vi "Init.vi"(8 "error in (no error)":errorcluster, 9 "Config File Path":path=path "", 10 "Name":string, 11 "Base In":refnum<class "Base.lvclass">) -> (0 "error out":errorcluster, 3 "Base Out":refnum<class "Base.lvclass">)   [LabVIEW 2020, in "Base.lvclass"]
doc: "Initialize the class and creates necessary references. Anything initialized here is released in the Clear.vi method."
uses:
  Base.lvclass
  Base.lvclass/Base.ctl
  <vilib>/Utility/file.llb/Application Directory.vi
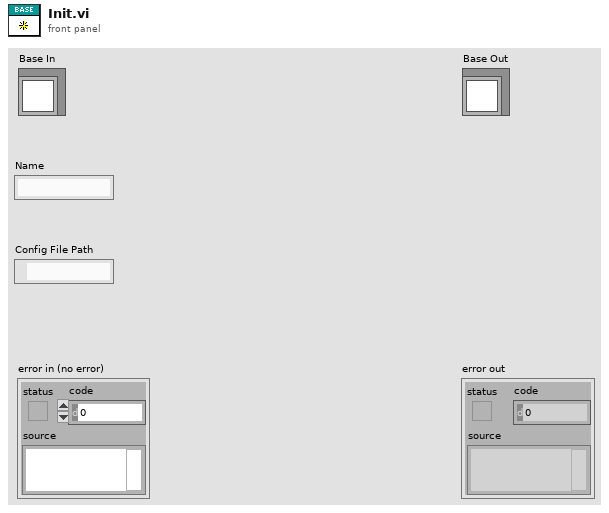
[diagram p1: front panel]
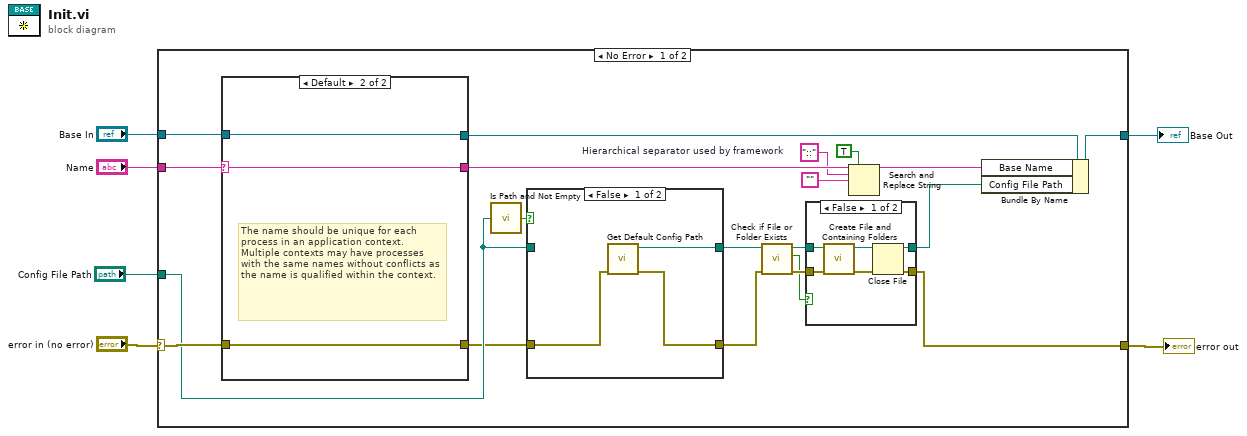
[diagram p0: block diagram]
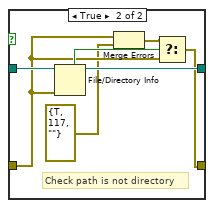
[diagram p3: hidden frame]
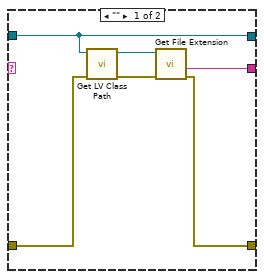
[diagram p4: hidden frame]
diagram:
  n1 = case shown="No Error" "error in (no error)" {
    selector: "error in (no error)" -> [w22 w54]
    tunnel: [w26 w55] -> w6
    tunnel: "Base In" -> [w25 w55]
    tunnel: "Name" -> [w23 _]
    tunnel: "Config File Path" -> [w20 _]
    tunnel: [w13 w54] -> w1
    frame No Error {
      w8 = "::"  # Hierarchical separator used by framework
      n2 = case shown="Default" w23 {
        selector: w23 -> [_ w51]
        tunnel: [w46 w51] -> w11
        tunnel: w25 -> [w45 w53]
        tunnel: w22 -> [w48 w52]
        tunnel: [w47 w52] -> w19
        tunnel: [w45 w53] -> w24
        frame "" {
          n3 = call <vilib>:"Get LV Class Path.vi"("error in (no error)"=w48, "object"=w45) -> ("error out"=w49:errorcluster, "class path"=w50:path)  [unwired: 8 in]
          n4 = call <vilib>:"Get File Extension.vi"("error in (no error)"=w49, "file"=w50) -> ("error out"=w47:errorcluster, "filename without extension"=w46:string)  [unwired: 5 in, 3 out]
        }
        frame Default {
          # "The name should be unique for each process in an application context. Multiple contexts may have processes with the same names without conflicts as the name is qualified within the context."
        }
      }
      n5 = call <vilib>:"Is Path and Not Empty.vi"("path"=w20) -> ("Is Path and Not Empty?"=w21:bool)  [unwired: 4 in]
      n6 = case shown="False" w21 {
        tunnel: w19 -> [w37 w39]
        tunnel: [w36 w42] -> w14
        tunnel: [w35 w44] -> w16
        tunnel: w20 -> [_ w43]
        frame False {
          n7 = call "Get Default Config Path.vi"("error in (no error)"=w37) -> ("error out"=w36:errorcluster, "appended path"=w35:path)  [unwired: 9 in]
        }
        frame True {
          # "Check path is not directory"
          n8 = File/Directory Info(path=w43, error in=w39) -> (path out=w44:path, directory=w41:bool)  [unwired: 5 out]
          n9 = Merge Errors(w39, errorcluster {"status"=TRUE, "code"=117, "source"=""} ("error out")) -> (w40:errorcluster)
          n10 = Select(t=w40, s=w41, f=w39) -> (s? t:f=w42:errorcluster)
        }
      }
      n11 = call <vilib>:"Check if File or Folder Exists.vi"("error in (no error)"=w14, "path"=w16) -> ("error out"=w17:errorcluster, "file or folder exists?"=w12:bool, "dup path"=w18:path)  [unwired: 7 in]
      n12 = case shown="False" w12 {
        tunnel: w18 -> [w30 w34]
        tunnel: w17 -> [w29 w33]
        tunnel: [w28 w34] -> w15
        tunnel: [w27 w33] -> w13
        frame False {
          n13 = call <vilib>:"Create File and Containing Folders.vi"("error in (no error)"=w29, "file path"=w30) -> ("error out"=w32:errorcluster, "refnum out"=w31:refnum<file>)  [unwired: 8 in]
          n14 = Close File(refnum=w31, error in=w32) -> (path=w28:path, error out=w27:errorcluster)
        }
        frame True {
        }
      }
      n15 = Search and Replace String(replace all?=TRUE ("replace all? (F)"), input string=w11, search string=w8, replace string="") -> (result string=w10:string)  [unwired: 4 in, 3 out]
      n16 = Bundle By Name(cluster=w24, "Base Name"=w10, "Config File Path"=w15) -> (w26:refnum<class "Base.lvclass">)
    }
    frame Error {
    }
  }
  "error out" <- w1
  "Base Out" <- w6
